vi "Control Mode Write Array.vi"(8 "error in":errorcluster, 9 "Channel Index":i32, 10 "Control Mode STS":u16, 11 "Chiller In":refnum<class "Chiller.lvclass">) -> (0 "error out":errorcluster, 3 "Chiller out":refnum<class "Chiller.lvclass">)   [LabVIEW 2023, in "Chiller.lvclass"]
uses:
  Chiller.lvclass
  Chiller.lvclass/Chiller.ctl
  Low Level Capabilities/Control Mode/Control Mode.lvclass
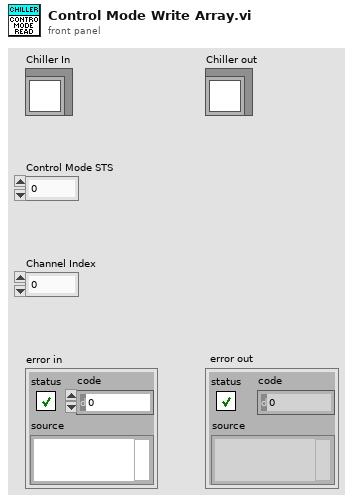
[diagram p1: front panel]
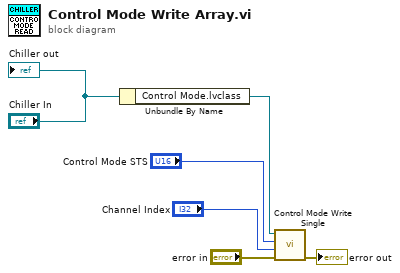
[diagram p0: block diagram]
diagram:
  n1 = Unbundle By Name("Chiller In") -> ("Control Mode.lvclass"=w1:refnum<class "Control Mode.lvclass">)
  n2 = call-dynamic "Control Mode Write Single.vi"("error in"="error in", "Channel Index"="Channel Index", "Control Mode STS"="Control Mode STS", "Control Mode in"=w1) -> ("error out"=→"error out":errorcluster)  [unwired: 6 in, 1 out]
  "Chiller out" <- "Chiller In"
